vi "ATSh_SetTriggerTimeOut.vi"(10 "TimeoutCount":u32, 11 "Handle":u32) -> (0 "Return Code":u32, 3 "Handle_Out":u32)   [LabVIEW 2010]
doc: "_____AlazarTech, Scope_____\n\nConfigure the Trigger TimeOut circuitry.\nHandle input.\n\nMaximum Timeout count is: 360 000 000 count x 10us = 1hour\nIf set to 0 ==> timeout infinite"
uses:
  ATSApi.dll
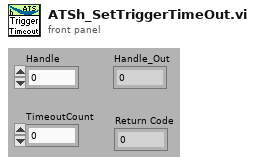
[diagram p1: front panel]
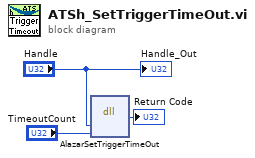
[diagram p0: block diagram]
diagram:
  n1 = dll-call lib="ATSApi.dll" fn="AlazarSetTriggerTimeOut"("h"="Handle", "Timeout"="TimeoutCount") -> (→"Return Code":u32)  [unwired: 5 in, 2 out]
  "Handle_Out" <- "Handle"
